vi "FTW-Connector-QueryActorInstanceStatus.vi"(0 "FTW Actor Connector":T1, 5 "Timeout":i32=100 format="%dmsec", 11 "error in":errorcluster) -> (4 "FTW Actor Connector out":T1, 6 "Actor Status":string, 8 "Roundtrip Time":dbl format="%.6fsec", 15 "error out":errorcluster)   [LabVIEW 2015]
doc: "Performs a \"cold call\" to connect to a running Actor Instance at the given Instance Inbox Address. Normally, this method is wrapped by a \"Construct\" method in each specific Actor Connector subclass."
uses:
  core/type/FTW-Type-Actor-Connector.ctl
  time/FTW-Time-RelativeTimer.vi
  error/FTW-ERR-ThrowError.vi
  reflection/FTW-Reflection-Type.vi
  error/FTW-ERR-NoErrorConstant.vi
  error/FTW-ERR-CallChain.vi
  string/FTW-STR-ReplaceWhitespace.vi
  reflection/FTW-Reflection-Array.vi
  reflection/FTW-Reflection-FTWObject.vi
  string/FTW-STR-Array-Delimit.vi
  lib/FTW-KernelFilepath.vi
  json/core/FTW-JSON-Core-EncodingFlags.vi
  codegen/xnode/json/fetch/FTW-JSON-Core-GetFlattenedValue.vi
  support/FTW-Socket-Core-LibraryError.vi
  actor/request/FTW-Request-InterpretResponse.vi
  codegen/xnode/FTW-Actor-Ask.xnode
  codegen/xnode/FTW-JSON-Fetch.xnode
panel:
  # "Inputs"
  # "Outputs"
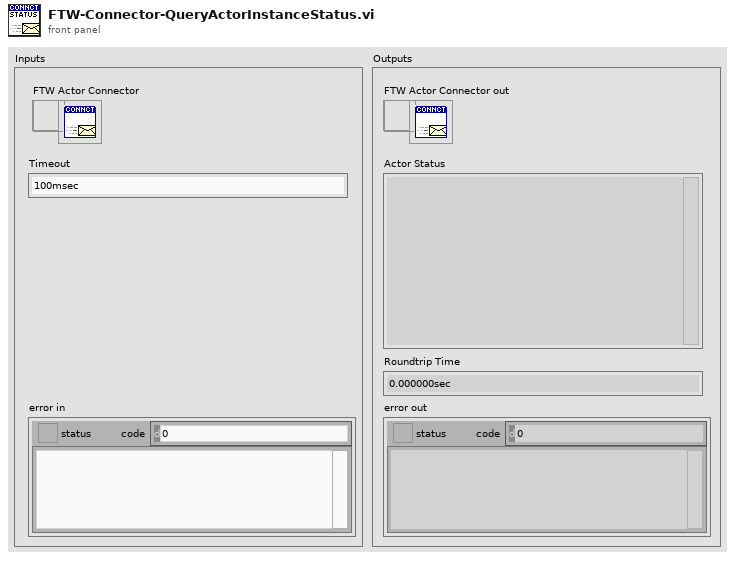
[diagram p1: front panel]
types:
  T1 = typedef "FTW-Type-Actor-Connector.ctl" = refnum<data-value>
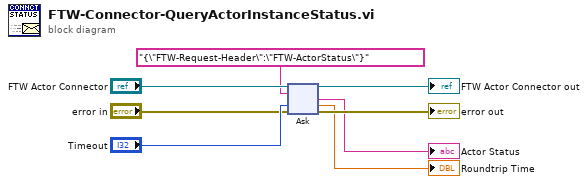
[diagram p0: block diagram]
diagram:
  n1 = xnode "Ask"("FTW Actor Connector"="FTW Actor Connector", "Request"="{\"FTW-Request-Header\":\"FTW-ActorStatus\"}", "Timeout"="Timeout", "error in"="error in") -> ("FTW Actor Connector out"=→"FTW Actor Connector out":T1, "Response"=→"Actor Status":string, "Roundtrip Time"=→"Roundtrip Time":dbl, "error out"=→"error out":errorcluster)  [unwired: 1 in]
